vi "_Parse ES Flatness Segment Result.vi"(8 "error in (no error)":errorcluster, 10 "Input String":string, 11 "VISA resource name":refnum<visa-resource-name>) -> (0 "error out":errorcluster, 1 "Results":T2 {"Max R2" format="%^.3e"; "Min R2" format="%^.3e"; "Max R1" format="%^.3e"; "Min R1" format="%^.3e"; "Max R2 Min R1" format="%^.3e"; "Max R1 Min R2" format="%^.3e"; "Ripple 2" format="%^.3e"; "Ripple 1" format="%^.3e"}, 2 "Reliability Results":T1, 3 "VISA resource name out":refnum<visa-resource-name>, 5 "Out Of Tolerance":i32, 7 "Statistic Expired":i32)   [LabVIEW 2020, in "Rohde&Schwarz CMWXP NR FR1 Measurement.lvlib"]
uses:
  <instrlib>/Rohde&Schwarz CMWXP NR FR1 Measurement/Rohde&Schwarz CMWXP NR FR1 Measurement.lvlib
  <instrlib>/Rohde&Schwarz CMWXP NR FR1 Measurement/Private/_SegReliability.ctl
  <instrlib>/Rohde&Schwarz CMWXP NR FR1 Measurement/Private/rsidr_core.llb/rsidr_core.lvlib
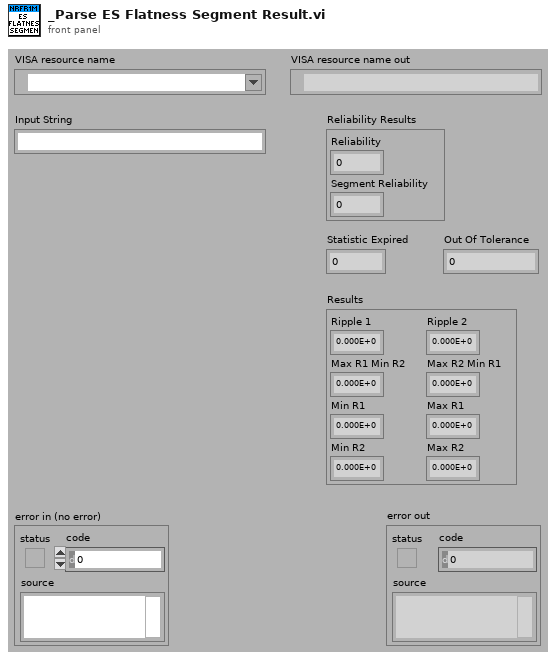
[diagram p1: front panel]
types:
  T1 = typedef "Rohde&Schwarz CMWXP NR FR1 Measurement.lvlib/_SegReliability.ctl" = cluster{"Reliability":i32, "Segment Reliability":i32}
  T2 = cluster{"Ripple 1":dbl, "Ripple 2":dbl, "Max R1 Min R2":dbl, "Max R2 Min R1":dbl, "Min R1":dbl, "Max R1":dbl, "Min R2":dbl, "Max R2":dbl}
  T3 = cluster{"double array out[0]":dbl, "double array out[1]":dbl, "double array out[2]":dbl, "double array out[3]":dbl, "double array out[4]":dbl, "double array out[5]":dbl, "double array out[6]":dbl, "double array out[7]":dbl}
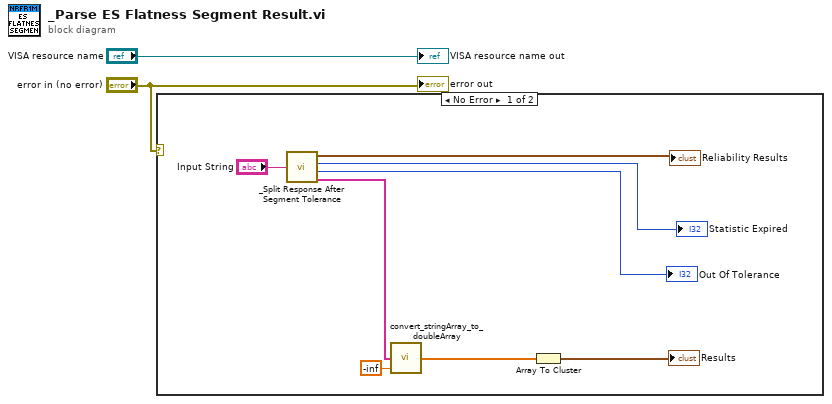
[diagram p0: block diagram]
diagram:
  n1 = case shown="No Error" "error in (no error)" {
    frame No Error {
      n2 = call <instrlib>:"_Split Response After Segment Tolerance.vi"("Input String"="Input String") -> ("Reliability Results"=→"Reliability Results":T1, "Statistic Expired"=→"Statistic Expired":i32, "Out Of Tolerance"=→"Out Of Tolerance":i32, "Response out"=w3:string[])
      n3 = call <instrlib>:"convert_stringArray_to_doubleArray.vi"("default (0)"=-inf, "string array in"=w3) -> ("double array out"=w8:dbl[])  [unwired: 3 in]
      n4 = Array To Cluster(array=w8) -> (cluster=→"Results":T3)
    }
    frame Error {
    }
  }
  "VISA resource name out" <- "VISA resource name"
  "error out" <- "error in (no error)"
